vi "Event Sent Data.vi"(8 "error in":errorcluster, 9 "EVENT Description":string) -> (0 "error out":errorcluster)   [LabVIEW 2023, in "HardwareAbstractionLayer_LVOOP.lvlib" / "Error Handler.lvclass"]
uses:
  Error Handler.lvclass
  Database/SQL Public VI/Control/DB Options.ctl
  Control/Error Data.ctl
  Control/Error_States.ctl
  Control/Error and Event Log.ctl
  <userlib>/_MGI/Application Control/MGI VI Reference/MGI Caller's VI Reference.vi
  Database/Database.lvclass
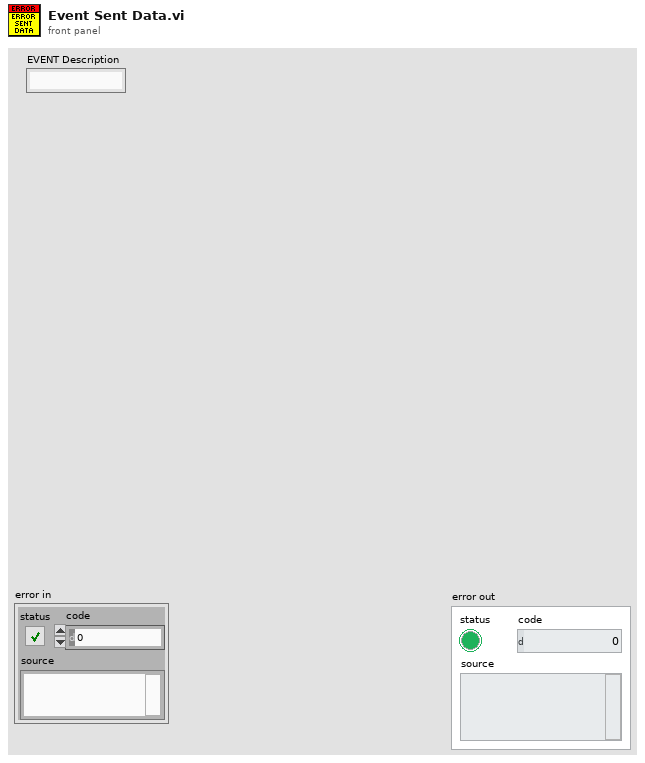
[diagram p1: front panel]
types:
  T1 = typedef "HardwareAbstractionLayer_LVOOP.lvlib/Database.lvclass/DB Options.ctl" = enum16{"Init", "Select Data", "Insert Data", "Update Data", "Delete Data", "Execute Query", "Create Schema", "Create Table", "List Tables", "List Columns", "Close"}
  T2 = typedef "HardwareAbstractionLayer_LVOOP.lvlib/Error Handler.lvclass/Error_States.ctl" = enum16{"No Error", "Error_Log", "Event_Log"}
  T3 = typedef "HardwareAbstractionLayer_LVOOP.lvlib/Error Handler.lvclass/Error and Event Log.ctl" = cluster{"Error/Event Log":string, "TimeStamp":string, "VI Source Name":string, "Description ":string}
  T4 = typedef "HardwareAbstractionLayer_LVOOP.lvlib/Error Handler.lvclass/Error Data.ctl" = cluster{"Data":variant, "States":T2}
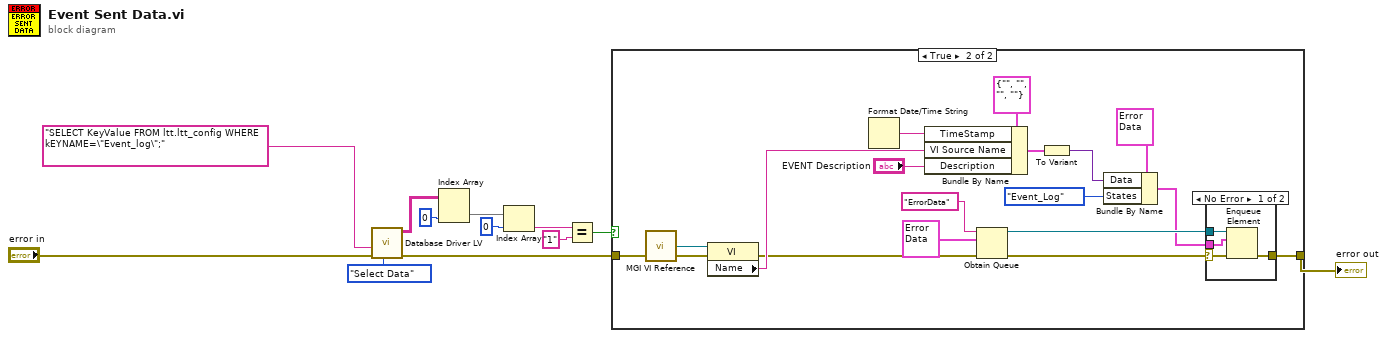
[diagram p0: block diagram]
diagram:
  n1 = call "Database Driver LV.vi"("Options"=DB_Options."Select Data", "error in"="error in", "SQL query"="SELECT KeyValue FROM ltt.ltt_config WHERE kEYNAME=\"Event_log\";") -> ("error out"=w6:errorcluster, "data"=w5:string[][])  [unwired: 5 in, 2 out]
  n2 = Index Array(array=w5, index (col)=0 ("disabled index (col)")) -> (element=w4:string[])  [unwired: 1 in]
  n3 = Index Array(array=w4, index=0) -> (element=w3:string)
  n4 = Equal?(x=w3, y="1") -> (x = y?=w1:bool)
  n5 = case shown="True" w1 {
    tunnel: [w13 w16] -> w12
    tunnel: w6 -> [w13 w15]
    frame False {
    }
    frame True {
      n6 = call-poly <userlib>:"MGI VI Reference.vi"() -> ("Caller's VI Reference"=w19:refnum<vi>)  [unwired: 1 in]
      n7 = property class="VI"(reference=w19, error in=w15) -> (error out=w20:errorcluster, "Name"=w21:string)  [unwired: 1 out]
      n8 = Format Date/Time String() -> (date/time string=w22:string)  [unwired: 3 in]
      n9 = Bundle By Name(cluster=T3 {"Error/Event Log"="", "TimeStamp"="", "VI Source Name"="", "Description "=""} ("Error and Event Log"), "TimeStamp"=w22, "VI Source Name"=w21, "Description"="EVENT Description") -> (w23:T3)
      n10 = Obtain Queue(name (unnamed)="ErrorData", element data type=T4 {"Data"=variant, "States"=enum."Event_Log"} ("Data"), error in (no error)=w20) -> (queue out=w28:refnum<queue>, error out=w27:errorcluster)  [unwired: 2 in, 1 out]
      n11 = To Variant(anything=w23) -> (Variant=w24:variant)
      n12 = Bundle By Name(cluster=T4 {"Data"=variant, "States"=enum."Event_Log"} ("Error and Event Data"), "Data"=w24, "States"=Error_States."Event_Log") -> (w25:T4)
      n13 = case shown="No Error" w27 {
        selector: w27 -> [w33 w35]
        tunnel: w28 -> [w34 _]
        tunnel: w25 -> [w32 _]
        tunnel: [w31 w35] -> w16
        frame No Error {
          n14 = Enqueue Element(queue=w34, element=w32, error in (no error)=w33) -> (error out=w31:errorcluster)  [unwired: 1 in, 2 out]
        }
        frame Error {
        }
      }
    }
  }
  "error out" <- w12
